vi "Variant To Byte Stream.vi"(8 "error in (no error)":errorcluster, 11 "data in":variant) -> (0 "error out":errorcluster, 1 "columns":i32, 2 "rows":i32, 3 "binary data out":u8[](array[numeric]), 5 "type":T1)   [LabVIEW 2020, in "GOLPI library.lvlib"]
doc: "Converts scalar, 1D or 2D input data to byte series in little endian."
uses:
  GOLPI library.lvlib
  <vilib>/Utility/Data Type/NI_Data Type.lvlib
  <vilib>/ErrorRing/Error Ring.xnode
  <vilib>/Utility/error.llb/Error Cluster From Error Code.vi
  <vilib>/Utility/Data Type/Type Definitions/Data Type.ctl
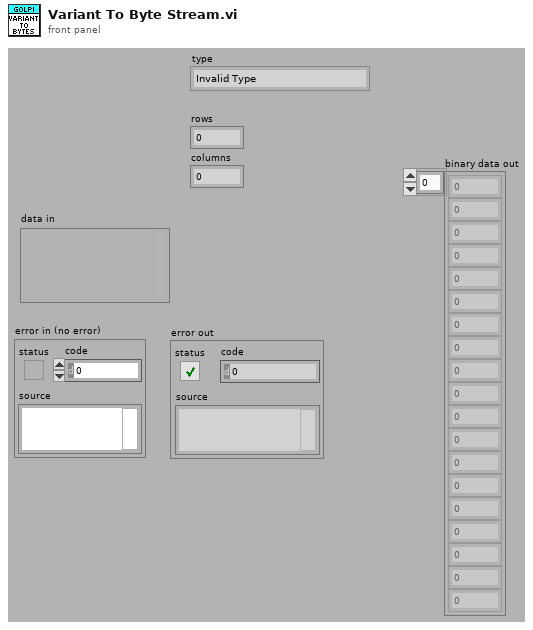
[diagram p1: front panel]
types:
  T1 = typedef "NI_Data Type.lvlib/Data Type.ctl" = enum8{"Invalid Type", "Void", "I8", "I16", "I32", "I64", "U8", "U16", "U32", "U64", "Single Float", "Double Float", "Extended Float", "Single Complex", "Double Complex", "Extended Complex", "Enum U8", "Enum U16", "Enum U32", "Enum U64", "Single Float With Unit", "Double Float With Unit", "Extended Float With Unit", "Single Complex with Unit", "Double Complex with Unit", "Extended Complex with Unit", "Boolean", "String", "Path", "Picture", "Tag", "Array", "Cluster", "Variant", "LV Variant", "Waveform", "Timestamp", "Digital Waveform", "Digital Data", "ExpressData", "Refnum", "External Data", "VI", "Poly VI", "LabVIEW Class Instance", "Fixed Point", "Set Collection", "Map Collection"}
  T2 = enum16{"big-endian, network order", "native, host order", "little-endian"}
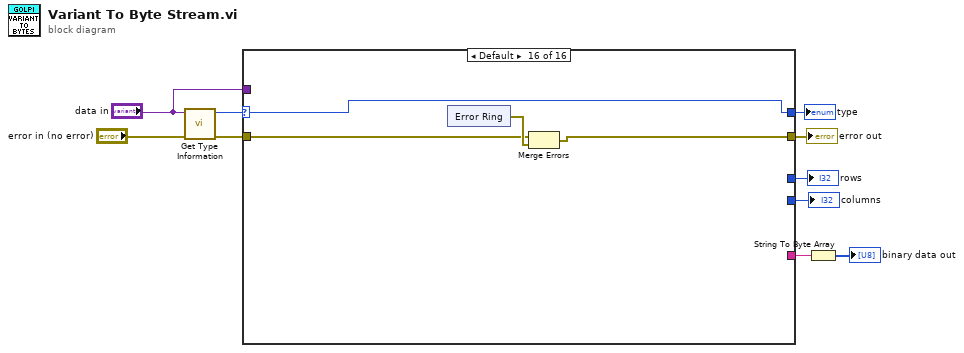
[diagram p0: block diagram]
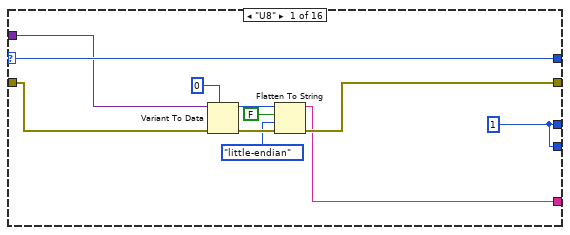
[diagram p2: hidden frame]
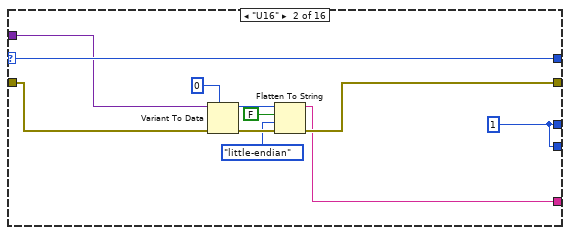
[diagram p3: hidden frame]
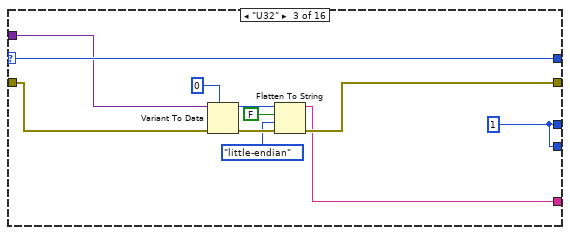
[diagram p4: hidden frame]
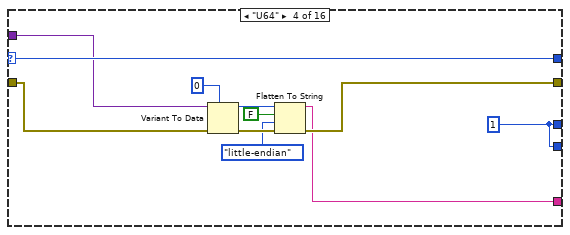
[diagram p5: hidden frame]
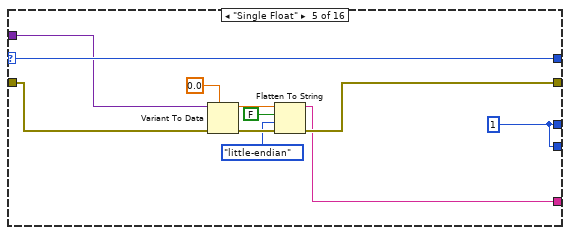
[diagram p6: hidden frame]
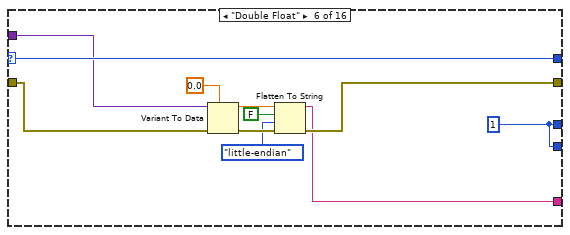
[diagram p7: hidden frame]
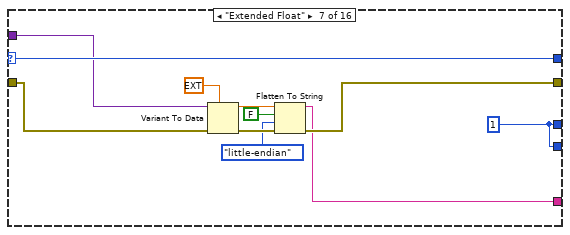
[diagram p8: hidden frame]
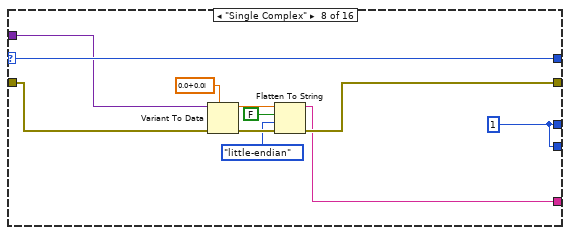
[diagram p9: hidden frame]
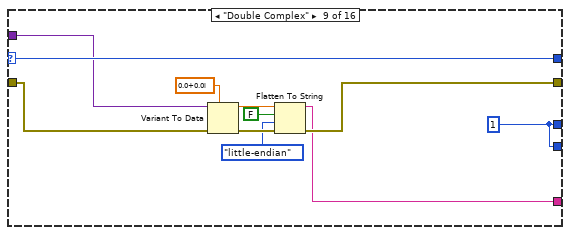
[diagram p10: hidden frame]
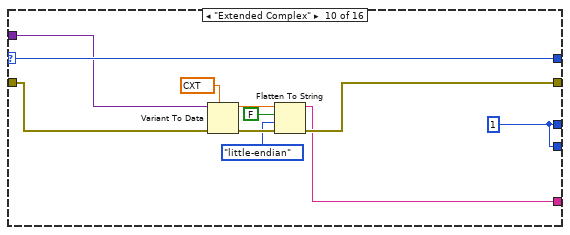
[diagram p11: hidden frame]
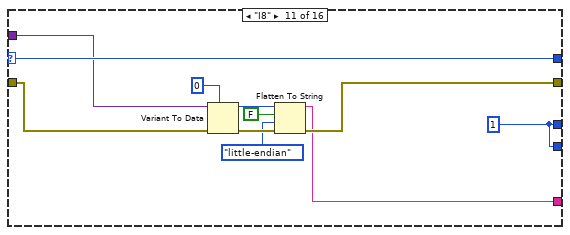
[diagram p12: hidden frame]
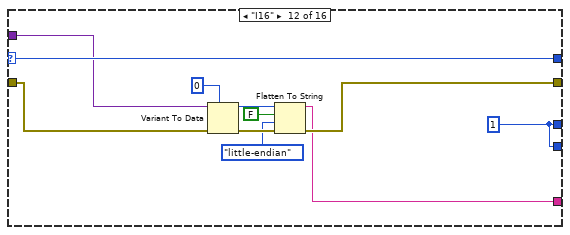
[diagram p13: hidden frame]
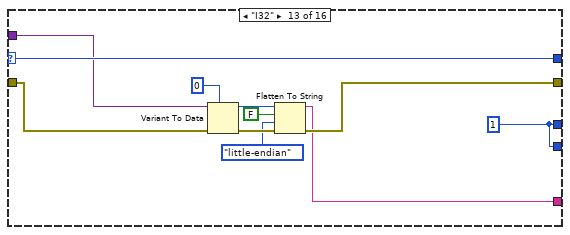
[diagram p14: hidden frame]
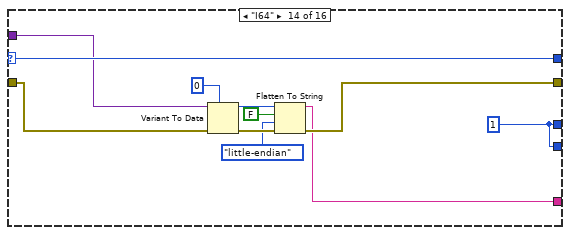
[diagram p15: hidden frame]
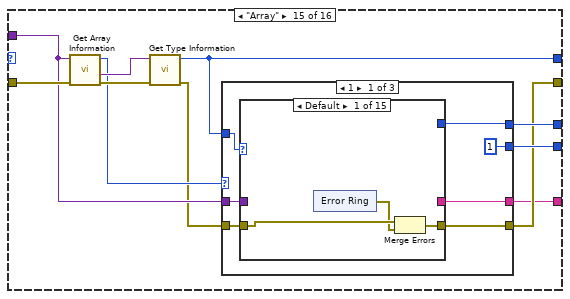
[diagram p16: hidden frame]
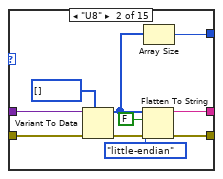
[diagram p17: hidden frame]
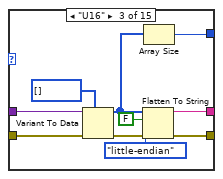
[diagram p18: hidden frame]
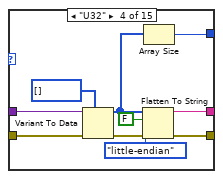
[diagram p19: hidden frame]
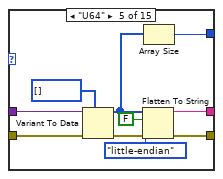
[diagram p20: hidden frame]
diagram:
  n1 = call <vilib>:"Get Type Information.vi"("error in (no error)"="error in (no error)", "variant"="data in") -> ("error out"=w9:errorcluster, "type"=w10:T1)  [unwired: 5 in, 3 out]
  n2 = case shown="Default" w10 {
    selector: w10 -> [w21 w32 w43 w54 w65 w76 w87 w98 w109 w120 w131 w142 w153 w164 _ w507]
    tunnel: w9 -> [w13 w24 w35 w46 w57 w68 w79 w90 w101 w112 w123 w134 w145 w156 w175 w509]
    tunnel: "data in" -> [w14 w25 w36 w47 w58 w69 w80 w91 w102 w113 w124 w135 w146 w157 w171 _]
    tunnel: [w21 w32 w43 w54 w65 w76 w87 w98 w109 w120 w131 w142 w153 w164 w166 w507] -> w3
    tunnel: [w20 w31 w42 w53 w64 w75 w86 w97 w108 w119 w130 w141 w152 w163 w169 _] -> w8
    tunnel: [w20 w31 w42 w53 w64 w75 w86 w97 w108 w119 w130 w141 w152 w163 w168 _] -> w7
    tunnel: [w12 w23 w34 w45 w56 w67 w78 w89 w100 w111 w122 w133 w144 w155 w167 w508] -> w5
    tunnel: [w11 w22 w33 w44 w55 w66 w77 w88 w99 w110 w121 w132 w143 w154 w165 _] -> w6
    frame "U8" {
      w20 = 1
      n3 = Variant To Data(error in=w13, type=u8 0, Variant=w14) -> (data=w15:u8, error out=w19:errorcluster)
      n4 = Flatten To String(anything=w15, prepend array or string size? (T)=FALSE, byte order (0:big-endian, network order)=T2."little-endian", error in (no error)=w19) -> (data string=w11:string, error out=w12:errorcluster)  [unwired: 1 out]
    }
    frame "U16" {
      w31 = 1
      n5 = Variant To Data(error in=w24, type=u16 0, Variant=w25) -> (data=w26:u16, error out=w30:errorcluster)
      n6 = Flatten To String(anything=w26, prepend array or string size? (T)=FALSE, byte order (0:big-endian, network order)=T2."little-endian", error in (no error)=w30) -> (data string=w22:string, error out=w23:errorcluster)  [unwired: 1 out]
    }
    frame "U32" {
      w42 = 1
      n7 = Variant To Data(error in=w35, type=u32 0, Variant=w36) -> (data=w37:u32, error out=w41:errorcluster)
      n8 = Flatten To String(anything=w37, prepend array or string size? (T)=FALSE, byte order (0:big-endian, network order)=T2."little-endian", error in (no error)=w41) -> (data string=w33:string, error out=w34:errorcluster)  [unwired: 1 out]
    }
    frame "U64" {
      w53 = 1
      n9 = Variant To Data(error in=w46, type=u64 0, Variant=w47) -> (data=w48:u64, error out=w52:errorcluster)
      n10 = Flatten To String(anything=w48, prepend array or string size? (T)=FALSE, byte order (0:big-endian, network order)=T2."little-endian", error in (no error)=w52) -> (data string=w44:string, error out=w45:errorcluster)  [unwired: 1 out]
    }
    frame "Single Float" {
      w64 = 1
      n11 = Variant To Data(error in=w57, type=sgl 0.0, Variant=w58) -> (data=w59:sgl, error out=w63:errorcluster)
      n12 = Flatten To String(anything=w59, prepend array or string size? (T)=FALSE, byte order (0:big-endian, network order)=T2."little-endian", error in (no error)=w63) -> (data string=w55:string, error out=w56:errorcluster)  [unwired: 1 out]
    }
    frame "Double Float" {
      w75 = 1
      n13 = Variant To Data(error in=w68, type=0.0, Variant=w69) -> (data=w70:dbl, error out=w74:errorcluster)
      n14 = Flatten To String(anything=w70, prepend array or string size? (T)=FALSE, byte order (0:big-endian, network order)=T2."little-endian", error in (no error)=w74) -> (data string=w66:string, error out=w67:errorcluster)  [unwired: 1 out]
    }
    frame "Extended Float" {
      w86 = 1
      n15 = Variant To Data(error in=w79, type=ext 0.0, Variant=w80) -> (data=w81:ext, error out=w85:errorcluster)
      n16 = Flatten To String(anything=w81, prepend array or string size? (T)=FALSE, byte order (0:big-endian, network order)=T2."little-endian", error in (no error)=w85) -> (data string=w77:string, error out=w78:errorcluster)  [unwired: 1 out]
    }
    frame "Single Complex" {
      w97 = 1
      n17 = Variant To Data(error in=w90, type=csg 0.0+0.0i, Variant=w91) -> (data=w92:csg, error out=w96:errorcluster)
      n18 = Flatten To String(anything=w92, prepend array or string size? (T)=FALSE, byte order (0:big-endian, network order)=T2."little-endian", error in (no error)=w96) -> (data string=w88:string, error out=w89:errorcluster)  [unwired: 1 out]
    }
    frame "Double Complex" {
      w108 = 1
      n19 = Variant To Data(error in=w101, type=cdb 0.0+0.0i, Variant=w102) -> (data=w103:cdb, error out=w107:errorcluster)
      n20 = Flatten To String(anything=w103, prepend array or string size? (T)=FALSE, byte order (0:big-endian, network order)=T2."little-endian", error in (no error)=w107) -> (data string=w99:string, error out=w100:errorcluster)  [unwired: 1 out]
    }
    frame "Extended Complex" {
      w119 = 1
      n21 = Variant To Data(error in=w112, type=cxt 0.0+0.0i, Variant=w113) -> (data=w114:cxt, error out=w118:errorcluster)
      n22 = Flatten To String(anything=w114, prepend array or string size? (T)=FALSE, byte order (0:big-endian, network order)=T2."little-endian", error in (no error)=w118) -> (data string=w110:string, error out=w111:errorcluster)  [unwired: 1 out]
    }
    frame "I8" {
      w130 = 1
      n23 = Variant To Data(error in=w123, type=i8 0, Variant=w124) -> (data=w125:i8, error out=w129:errorcluster)
      n24 = Flatten To String(anything=w125, prepend array or string size? (T)=FALSE, byte order (0:big-endian, network order)=T2."little-endian", error in (no error)=w129) -> (data string=w121:string, error out=w122:errorcluster)  [unwired: 1 out]
    }
    frame "I16" {
      w141 = 1
      n25 = Variant To Data(error in=w134, type=i16 0, Variant=w135) -> (data=w136:i16, error out=w140:errorcluster)
      n26 = Flatten To String(anything=w136, prepend array or string size? (T)=FALSE, byte order (0:big-endian, network order)=T2."little-endian", error in (no error)=w140) -> (data string=w132:string, error out=w133:errorcluster)  [unwired: 1 out]
    }
    frame "I32" {
      w152 = 1
      n27 = Variant To Data(error in=w145, type=0, Variant=w146) -> (data=w147:i32, error out=w151:errorcluster)
      n28 = Flatten To String(anything=w147, prepend array or string size? (T)=FALSE, byte order (0:big-endian, network order)=T2."little-endian", error in (no error)=w151) -> (data string=w143:string, error out=w144:errorcluster)  [unwired: 1 out]
    }
    frame "I64" {
      w163 = 1
      n29 = Variant To Data(error in=w156, type=i64 0, Variant=w157) -> (data=w158:i64, error out=w162:errorcluster)
      n30 = Flatten To String(anything=w158, prepend array or string size? (T)=FALSE, byte order (0:big-endian, network order)=T2."little-endian", error in (no error)=w162) -> (data string=w154:string, error out=w155:errorcluster)  [unwired: 1 out]
    }
    frame "Array" {
      n31 = call <vilib>:"Get Array Information.vi"("error in (no error)"=w175, "variant"=w171) -> ("error out"=w174:errorcluster, "array element data type"=w173:variant, "number of dimensions"=w172:i32)  [unwired: 6 in, 1 out]
      n32 = call <vilib>:"Get Type Information.vi"("error in (no error)"=w174, "variant"=w173) -> ("error out"=w170:errorcluster, "type"=w166:T1)  [unwired: 5 in, 3 out]
      n33 = case shown="1" w172 {
        tunnel: w171 -> [w182 w338 _]
        tunnel: w170 -> [w181 w337 _]
        tunnel: [w180 w336 w501] -> w167
        tunnel: [w176 w334 _] -> w169
        tunnel: [1 w333 _] -> w168
        tunnel: w166 -> [w178 w332 _]
        tunnel: [w177 w331 _] -> w165
        frame 1 {
          n34 = case shown="Default" w178 {
            tunnel: w182 -> [_ w199 w209 w219 w229 w239 w249 w259 w269 w279 w289 w299 w309 w319 w329]
            tunnel: w181 -> [w184 w198 w208 w218 w228 w238 w248 w258 w268 w278 w288 w298 w308 w318 w328]
            tunnel: [w185 w196 w206 w216 w226 w236 w246 w256 w266 w276 w286 w296 w306 w316 w326] -> w180
            tunnel: [_ w192 w202 w212 w222 w232 w242 w252 w262 w272 w282 w292 w302 w312 w322] -> w177
            tunnel: [_ w191 w201 w211 w221 w231 w241 w251 w261 w271 w281 w291 w301 w311 w321] -> w176
            frame Default {
              n35 = xnode "Error Ring"() -> ("error out"=w183:errorcluster)
              n36 = Merge Errors(w184, w183) -> (w185:errorcluster)
            }
            frame "U8" {
              n37 = Variant To Data(error in=w198, type=u8[] [], Variant=w199) -> (data=w195:u8[], error out=w197:errorcluster)
              n38 = Flatten To String(anything=w195, prepend array or string size? (T)=FALSE, byte order (0:big-endian, network order)=T2."little-endian", error in (no error)=w197) -> (data string=w192:string, error out=w196:errorcluster)  [unwired: 1 out]
              n39 = Array Size(array=w195) -> (size(s)=w191:i32)
            }
            frame "U16" {
              n40 = Variant To Data(error in=w208, type=u16[] [], Variant=w209) -> (data=w205:u16[], error out=w207:errorcluster)
              n41 = Flatten To String(anything=w205, prepend array or string size? (T)=FALSE, byte order (0:big-endian, network order)=T2."little-endian", error in (no error)=w207) -> (data string=w202:string, error out=w206:errorcluster)  [unwired: 1 out]
              n42 = Array Size(array=w205) -> (size(s)=w201:i32)
            }
            frame "U32" {
              n43 = Variant To Data(error in=w218, type=u32[] [], Variant=w219) -> (data=w215:u32[], error out=w217:errorcluster)
              n44 = Flatten To String(anything=w215, prepend array or string size? (T)=FALSE, byte order (0:big-endian, network order)=T2."little-endian", error in (no error)=w217) -> (data string=w212:string, error out=w216:errorcluster)  [unwired: 1 out]
              n45 = Array Size(array=w215) -> (size(s)=w211:i32)
            }
            frame "U64" {
              n46 = Variant To Data(error in=w228, type=u64[] [], Variant=w229) -> (data=w225:u64[], error out=w227:errorcluster)
              n47 = Flatten To String(anything=w225, prepend array or string size? (T)=FALSE, byte order (0:big-endian, network order)=T2."little-endian", error in (no error)=w227) -> (data string=w222:string, error out=w226:errorcluster)  [unwired: 1 out]
              n48 = Array Size(array=w225) -> (size(s)=w221:i32)
            }
            frame "Single Float" {
              n49 = Variant To Data(error in=w238, type=sgl[] [], Variant=w239) -> (data=w235:sgl[], error out=w237:errorcluster)
              n50 = Flatten To String(anything=w235, prepend array or string size? (T)=FALSE, byte order (0:big-endian, network order)=T2."little-endian", error in (no error)=w237) -> (data string=w232:string, error out=w236:errorcluster)  [unwired: 1 out]
              n51 = Array Size(array=w235) -> (size(s)=w231:i32)
            }
            frame "Double Float" {
              n52 = Variant To Data(error in=w248, type=dbl[] [], Variant=w249) -> (data=w245:dbl[], error out=w247:errorcluster)
              n53 = Flatten To String(anything=w245, prepend array or string size? (T)=FALSE, byte order (0:big-endian, network order)=T2."little-endian", error in (no error)=w247) -> (data string=w242:string, error out=w246:errorcluster)  [unwired: 1 out]
              n54 = Array Size(array=w245) -> (size(s)=w241:i32)
            }
            frame "Extended Float" {
              n55 = Variant To Data(error in=w258, type=ext[] [], Variant=w259) -> (data=w255:ext[], error out=w257:errorcluster)
              n56 = Flatten To String(anything=w255, prepend array or string size? (T)=FALSE, byte order (0:big-endian, network order)=T2."little-endian", error in (no error)=w257) -> (data string=w252:string, error out=w256:errorcluster)  [unwired: 1 out]
              n57 = Array Size(array=w255) -> (size(s)=w251:i32)
            }
            frame "Single Complex" {
              n58 = Variant To Data(error in=w268, type=csg[] [], Variant=w269) -> (data=w265:csg[], error out=w267:errorcluster)
              n59 = Flatten To String(anything=w265, prepend array or string size? (T)=FALSE, byte order (0:big-endian, network order)=T2."little-endian", error in (no error)=w267) -> (data string=w262:string, error out=w266:errorcluster)  [unwired: 1 out]
              n60 = Array Size(array=w265) -> (size(s)=w261:i32)
            }
            frame "Double Complex" {
              n61 = Variant To Data(error in=w278, type=cdb[] [], Variant=w279) -> (data=w275:cdb[], error out=w277:errorcluster)
              n62 = Flatten To String(anything=w275, prepend array or string size? (T)=FALSE, byte order (0:big-endian, network order)=T2."little-endian", error in (no error)=w277) -> (data string=w272:string, error out=w276:errorcluster)  [unwired: 1 out]
              n63 = Array Size(array=w275) -> (size(s)=w271:i32)
            }
            frame "Extended Complex" {
              n64 = Variant To Data(error in=w288, type=cxt[] [], Variant=w289) -> (data=w285:cxt[], error out=w287:errorcluster)
              n65 = Flatten To String(anything=w285, prepend array or string size? (T)=FALSE, byte order (0:big-endian, network order)=T2."little-endian", error in (no error)=w287) -> (data string=w282:string, error out=w286:errorcluster)  [unwired: 1 out]
              n66 = Array Size(array=w285) -> (size(s)=w281:i32)
            }
            frame "I8" {
              n67 = Variant To Data(error in=w298, type=i8[] [], Variant=w299) -> (data=w295:i8[], error out=w297:errorcluster)
              n68 = Flatten To String(anything=w295, prepend array or string size? (T)=FALSE, byte order (0:big-endian, network order)=T2."little-endian", error in (no error)=w297) -> (data string=w292:string, error out=w296:errorcluster)  [unwired: 1 out]
              n69 = Array Size(array=w295) -> (size(s)=w291:i32)
            }
            frame "I16" {
              n70 = Variant To Data(error in=w308, type=i16[] [], Variant=w309) -> (data=w305:i16[], error out=w307:errorcluster)
              n71 = Flatten To String(anything=w305, prepend array or string size? (T)=FALSE, byte order (0:big-endian, network order)=T2."little-endian", error in (no error)=w307) -> (data string=w302:string, error out=w306:errorcluster)  [unwired: 1 out]
              n72 = Array Size(array=w305) -> (size(s)=w301:i32)
            }
            frame "I32" {
              n73 = Variant To Data(error in=w318, type=i32[] [], Variant=w319) -> (data=w315:i32[], error out=w317:errorcluster)
              n74 = Flatten To String(anything=w315, prepend array or string size? (T)=FALSE, byte order (0:big-endian, network order)=T2."little-endian", error in (no error)=w317) -> (data string=w312:string, error out=w316:errorcluster)  [unwired: 1 out]
              n75 = Array Size(array=w315) -> (size(s)=w311:i32)
            }
            frame "I64" {
              n76 = Variant To Data(error in=w328, type=i64[] [], Variant=w329) -> (data=w325:i64[], error out=w327:errorcluster)
              n77 = Flatten To String(anything=w325, prepend array or string size? (T)=FALSE, byte order (0:big-endian, network order)=T2."little-endian", error in (no error)=w327) -> (data string=w322:string, error out=w326:errorcluster)  [unwired: 1 out]
              n78 = Array Size(array=w325) -> (size(s)=w321:i32)
            }
          }
        }
        frame 2 {
          n79 = case shown="\"I64\"" w332 {
            tunnel: w338 -> [_ w356 w367 w378 w389 w400 w411 w422 w433 w444 w455 w466 w477 w488 w499]
            tunnel: w337 -> [w340 w355 w366 w377 w388 w399 w410 w421 w432 w443 w454 w465 w476 w487 w498]
            tunnel: [w339 w349 w360 w371 w382 w393 w404 w415 w426 w437 w448 w459 w470 w481 w492] -> w336
            tunnel: [_ w354 w365 w376 w387 w398 w409 w420 w431 w442 w453 w464 w475 w486 w497] -> w335
            tunnel: [_ w348 w359 w370 w381 w392 w403 w414 w425 w436 w447 w458 w469 w480 w491] -> w331
            frame "Invalid Type", Default {
              n80 = xnode "Error Ring"() -> ("error out"=w341:errorcluster)
              n81 = Merge Errors(w340, w341) -> (w339:errorcluster)
            }
            frame "U8" {
              n82 = Variant To Data(error in=w355, type=u8[][] [], Variant=w356) -> (data=w350:u8[][], error out=w351:errorcluster)
              n83 = Transpose 2D Array(2D array=w350) -> (transposed array=w347:u8[][])
              n84 = Array Size(array=w350) -> (size(s)=w354:i32[])
              n85 = Flatten To String(anything=w347, prepend array or string size? (T)=FALSE, byte order (0:big-endian, network order)=T2."little-endian", error in (no error)=w351) -> (data string=w348:string, error out=w349:errorcluster)  [unwired: 1 out]
            }
            frame "U16" {
              n86 = Variant To Data(error in=w366, type=u16[][] [], Variant=w367) -> (data=w361:u16[][], error out=w362:errorcluster)
              n87 = Transpose 2D Array(2D array=w361) -> (transposed array=w358:u16[][])
              n88 = Array Size(array=w361) -> (size(s)=w365:i32[])
              n89 = Flatten To String(anything=w358, prepend array or string size? (T)=FALSE, byte order (0:big-endian, network order)=T2."little-endian", error in (no error)=w362) -> (data string=w359:string, error out=w360:errorcluster)  [unwired: 1 out]
            }
            frame "U32" {
              n90 = Variant To Data(error in=w377, type=u32[][] [], Variant=w378) -> (data=w372:u32[][], error out=w373:errorcluster)
              n91 = Transpose 2D Array(2D array=w372) -> (transposed array=w369:u32[][])
              n92 = Array Size(array=w372) -> (size(s)=w376:i32[])
              n93 = Flatten To String(anything=w369, prepend array or string size? (T)=FALSE, byte order (0:big-endian, network order)=T2."little-endian", error in (no error)=w373) -> (data string=w370:string, error out=w371:errorcluster)  [unwired: 1 out]
            }
            frame "U64" {
              n94 = Variant To Data(error in=w388, type=u64[][] [], Variant=w389) -> (data=w383:u64[][], error out=w384:errorcluster)
              n95 = Transpose 2D Array(2D array=w383) -> (transposed array=w380:u64[][])
              n96 = Array Size(array=w383) -> (size(s)=w387:i32[])
              n97 = Flatten To String(anything=w380, prepend array or string size? (T)=FALSE, byte order (0:big-endian, network order)=T2."little-endian", error in (no error)=w384) -> (data string=w381:string, error out=w382:errorcluster)  [unwired: 1 out]
            }
            frame "Single Float" {
              n98 = Variant To Data(error in=w399, type=sgl[][] [], Variant=w400) -> (data=w394:sgl[][], error out=w395:errorcluster)
              n99 = Transpose 2D Array(2D array=w394) -> (transposed array=w391:sgl[][])
              n100 = Array Size(array=w394) -> (size(s)=w398:i32[])
              n101 = Flatten To String(anything=w391, prepend array or string size? (T)=FALSE, byte order (0:big-endian, network order)=T2."little-endian", error in (no error)=w395) -> (data string=w392:string, error out=w393:errorcluster)  [unwired: 1 out]
            }
            frame "Double Float" {
              n102 = Variant To Data(error in=w410, type=dbl[][] [], Variant=w411) -> (data=w405:dbl[][], error out=w406:errorcluster)
              n103 = Transpose 2D Array(2D array=w405) -> (transposed array=w402:dbl[][])
              n104 = Array Size(array=w405) -> (size(s)=w409:i32[])
              n105 = Flatten To String(anything=w402, prepend array or string size? (T)=FALSE, byte order (0:big-endian, network order)=T2."little-endian", error in (no error)=w406) -> (data string=w403:string, error out=w404:errorcluster)  [unwired: 1 out]
            }
            frame "Extended Float" {
              n106 = Variant To Data(error in=w421, type=ext[][] [], Variant=w422) -> (data=w416:ext[][], error out=w417:errorcluster)
              n107 = Transpose 2D Array(2D array=w416) -> (transposed array=w413:ext[][])
              n108 = Array Size(array=w416) -> (size(s)=w420:i32[])
              n109 = Flatten To String(anything=w413, prepend array or string size? (T)=FALSE, byte order (0:big-endian, network order)=T2."little-endian", error in (no error)=w417) -> (data string=w414:string, error out=w415:errorcluster)  [unwired: 1 out]
            }
            frame "Single Complex" {
              n110 = Variant To Data(error in=w432, type=csg[][] [], Variant=w433) -> (data=w427:csg[][], error out=w428:errorcluster)
              n111 = Transpose 2D Array(2D array=w427) -> (transposed array=w424:csg[][])
              n112 = Array Size(array=w427) -> (size(s)=w431:i32[])
              n113 = Flatten To String(anything=w424, prepend array or string size? (T)=FALSE, byte order (0:big-endian, network order)=T2."little-endian", error in (no error)=w428) -> (data string=w425:string, error out=w426:errorcluster)  [unwired: 1 out]
            }
            frame "Double Complex" {
              n114 = Variant To Data(error in=w443, type=cdb[][] [], Variant=w444) -> (data=w438:cdb[][], error out=w439:errorcluster)
              n115 = Transpose 2D Array(2D array=w438) -> (transposed array=w435:cdb[][])
              n116 = Array Size(array=w438) -> (size(s)=w442:i32[])
              n117 = Flatten To String(anything=w435, prepend array or string size? (T)=FALSE, byte order (0:big-endian, network order)=T2."little-endian", error in (no error)=w439) -> (data string=w436:string, error out=w437:errorcluster)  [unwired: 1 out]
            }
            frame "Extended Complex" {
              n118 = Variant To Data(error in=w454, type=cxt[][] [], Variant=w455) -> (data=w449:cxt[][], error out=w450:errorcluster)
              n119 = Transpose 2D Array(2D array=w449) -> (transposed array=w446:cxt[][])
              n120 = Array Size(array=w449) -> (size(s)=w453:i32[])
              n121 = Flatten To String(anything=w446, prepend array or string size? (T)=FALSE, byte order (0:big-endian, network order)=T2."little-endian", error in (no error)=w450) -> (data string=w447:string, error out=w448:errorcluster)  [unwired: 1 out]
            }
            frame "I8" {
              n122 = Variant To Data(error in=w465, type=i8[][] [], Variant=w466) -> (data=w460:i8[][], error out=w461:errorcluster)
              n123 = Transpose 2D Array(2D array=w460) -> (transposed array=w457:i8[][])
              n124 = Array Size(array=w460) -> (size(s)=w464:i32[])
              n125 = Flatten To String(anything=w457, prepend array or string size? (T)=FALSE, byte order (0:big-endian, network order)=T2."little-endian", error in (no error)=w461) -> (data string=w458:string, error out=w459:errorcluster)  [unwired: 1 out]
            }
            frame "I16" {
              n126 = Variant To Data(error in=w476, type=i16[][] [], Variant=w477) -> (data=w471:i16[][], error out=w472:errorcluster)
              n127 = Transpose 2D Array(2D array=w471) -> (transposed array=w468:i16[][])
              n128 = Array Size(array=w471) -> (size(s)=w475:i32[])
              n129 = Flatten To String(anything=w468, prepend array or string size? (T)=FALSE, byte order (0:big-endian, network order)=T2."little-endian", error in (no error)=w472) -> (data string=w469:string, error out=w470:errorcluster)  [unwired: 1 out]
            }
            frame "I32" {
              n130 = Variant To Data(error in=w487, type=i32[][] [], Variant=w488) -> (data=w482:i32[][], error out=w483:errorcluster)
              n131 = Transpose 2D Array(2D array=w482) -> (transposed array=w479:i32[][])
              n132 = Array Size(array=w482) -> (size(s)=w486:i32[])
              n133 = Flatten To String(anything=w479, prepend array or string size? (T)=FALSE, byte order (0:big-endian, network order)=T2."little-endian", error in (no error)=w483) -> (data string=w480:string, error out=w481:errorcluster)  [unwired: 1 out]
            }
            frame "I64" {
              n134 = Variant To Data(error in=w498, type=i64[][] [], Variant=w499) -> (data=w493:i64[][], error out=w494:errorcluster)
              n135 = Transpose 2D Array(2D array=w493) -> (transposed array=w490:i64[][])
              n136 = Array Size(array=w493) -> (size(s)=w497:i32[])
              n137 = Flatten To String(anything=w490, prepend array or string size? (T)=FALSE, byte order (0:big-endian, network order)=T2."little-endian", error in (no error)=w494) -> (data string=w491:string, error out=w492:errorcluster)  [unwired: 1 out]
            }
          }
          n138 = Index Array(array=w335) -> (element #1=w334:i32, element #2=w333:i32)  [unwired: 2 in]
        }
        frame Default {
          n139 = xnode "Error Ring"() -> ("error out"=w501:errorcluster)
        }
      }
    }
    frame Default {
      n140 = xnode "Error Ring"() -> ("error out"=w510:errorcluster)
      n141 = Merge Errors(w509, w510) -> (w508:errorcluster)
    }
  }
  "rows" <- w8
  "columns" <- w7
  "error out" <- w5
  "type" <- w3
  n142 = String To Byte Array(string=w6) -> (unsigned byte array=→"binary data out":u8[])
